vi "software_id.vi"(6 "timeout (25000ms)":i32=25000, 8 "error in (no error)":errorcluster, 11 "daemon reference in":refnum<k5>) -> (0 "error out":errorcluster, 1 "component":string, 2 "project":string, 3 "daemon reference out":refnum<k5>, 5 "command out":string="software_id")   [LabVIEW 2017]
doc: "<b>Command: </b>\"software_id\"\n\n<b>Description: </b> Queries the target for the software ID which contains the Project and Component.\n\n<b>Parameters: </b> None\n____________________________________________\nDIPC 692 Daemon API 10.0.0.1\nSam Tee - Dyson Technology Ltd\nCopyright (c) 2024, Dyson Technology Ltd"
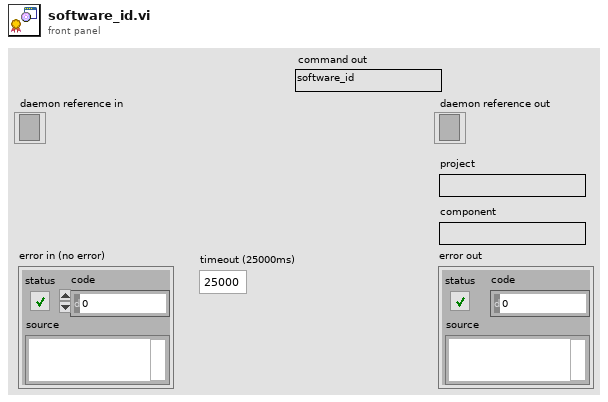
[diagram p1: front panel]
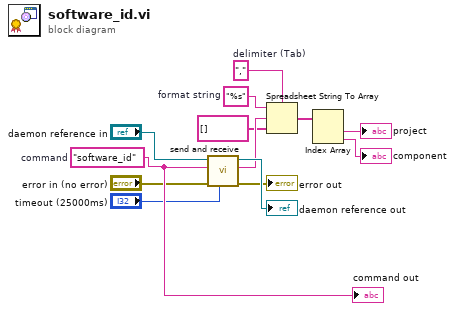
[diagram p0: block diagram]
diagram:
  w4 = ","  # delimiter (Tab)
  w5 = "%s"  # format string
  w11 = "software_id"  # command
  n1 = call "send and receive.vi"("timeout (25000ms)"="timeout (25000ms)", "error in (no error)"="error in (no error)", "command"=w11, "daemon reference in"="daemon reference in") -> ("error out"=→"error out":errorcluster, "response"=w7:string, "daemon reference out"=→"daemon reference out":refnum<k5>)  [unwired: 5 in]
  n2 = Spreadsheet String To Array(delimiter (Tab)=w4, format string=w5, spreadsheet string=w7, array type (2D Dbl)=string[] []) -> (array=w3:string[])
  n3 = Index Array(array=w3) -> (element #1=→"project":string, element #2=→"component":string)  [unwired: 2 in]
  "command out" <- w11
